vi "Clear_Info.vi"(8 "error in (no error)":errorcluster, 9 "index in":string, 10 "buildObject":T1) -> (0 "error out":errorcluster, 1 "index out":string, 2 "buildObject out":T1)   [LabVIEW 2020, in "IB_RegData.lvclass"]
uses:
  <vilib>/AppBuilder/IB_Classes/RegData/IB_RegData.lvclass
  <vilib>/AppBuilder/IB_Classes/RegData/IB_RegData.lvclass/IB_RegData.ctl
  <vilib>/AppBuilder/IB_RW_Project/IB_RW_Project_PropBag_Action.ctl
  <resource>/Framework/Providers/API/ItemRef.ctl
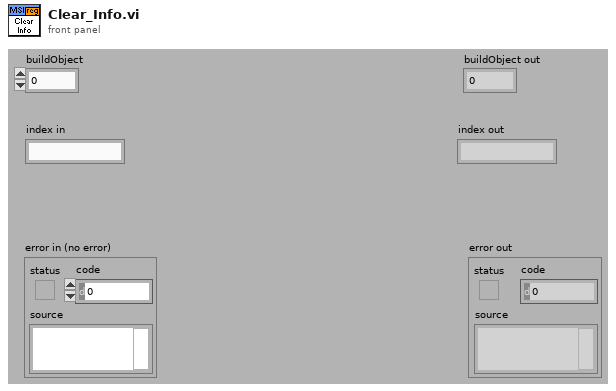
[diagram p1: front panel]
types:
  T1 = typedef "ItemRef.ctl" = u64
  T2 = typedef "IB_RW_Project_PropBag_Action.ctl" = enum16{"read", "write", "clear", "readPrevious", "writePrevious", "clearPrevious"}
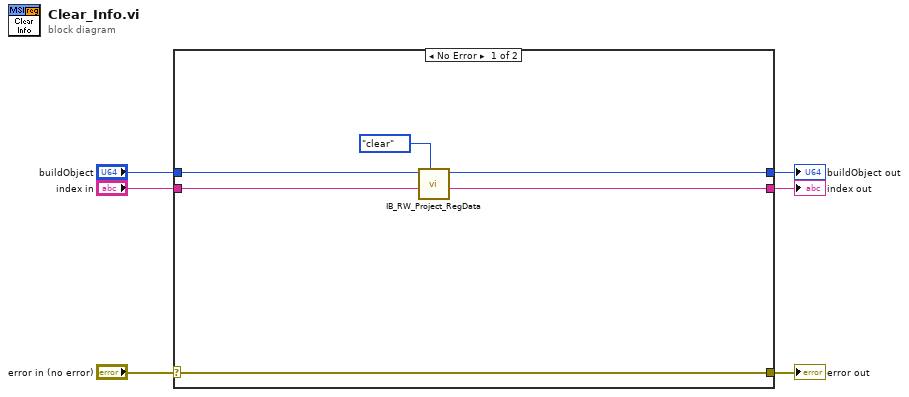
[diagram p0: block diagram]
diagram:
  n1 = case shown="No Error" "error in (no error)" {
    selector: "error in (no error)" -> [w12 w15]
    tunnel: [w12 w15] -> w5
    tunnel: "buildObject" -> [w9 w14]
    tunnel: [w11 w14] -> w3
    tunnel: "index in" -> [w8 w13]
    tunnel: [w7 w13] -> w1
    frame No Error {
      n2 = call <vilib>:"IB_RW_Project_RegData.vi"("action"=IB_RW_Project_PropBag_Action."clear", "index in"=w8, "buildObject"=w9) -> ("index out"=w7:string, "buildObject out"=w11:T1)  [unwired: 5 in, 2 out]
    }
    frame Error {
    }
  }
  "error out" <- w5
  "buildObject out" <- w3
  "index out" <- w1
